vi "read data.vi"() -> ()   [LabVIEW 2016]
uses:
  <vilib>/Utility/file.llb/Read Delimited Spreadsheet (string).vi
panel:
  in  "file path (dialog if empty)":path
  out "Waveform Chart":dbl(graph)
  in  "stop":bool
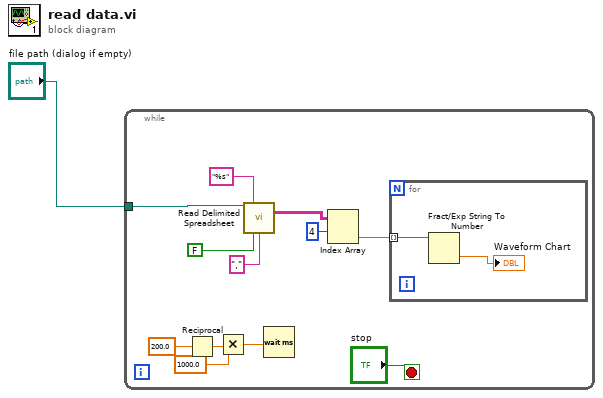
[diagram p0: block diagram]
diagram:
  n1 = while {
    tunnel: "file path (dialog if empty)" -> [w10]
    stop <- "stop" stop-if-true
    n2 = Reciprocal(x=200.0) -> (1/x=w8:dbl)
    n3 = Multiply(x=1000.0, y=w8) -> (x*y=w6:dbl)
    n4 = call-poly <vilib>:"Read Delimited Spreadsheet.vi"("file path (dialog if empty)"=w10, "format (%s)"="%s", "transpose? (F)"=FALSE ("transpose (no:F)"), "delimiter (\\t)"="," ("delimiter (\\t)")) -> ("all rows"=w4:string[][])  [unwired: 6 in, 5 out]
    n5 = Wait (ms)(milliseconds to wait=w6) -> ()  [unwired: 1 out]
    n6 = Index Array(array=w4, index (row)=4) -> (element=w2:string[])  [unwired: 1 in]
    n7 = for {
      tunnel: w2 -> [w15] mode=indexing
      n8 = Fract/Exp String To Number(string=w15) -> (number=→"Waveform Chart":dbl)  [unwired: 3 in, 1 out]
    }
  }
